vi "AH_ParseMSG.vi"(5 "InputMSG":string, 11 "error in (no error)":errorcluster) -> (2 "Cap Ind":string, 3 "Los Ind":string, 4 "Cap":dbl, 6 "Los":dbl, 8 "ExVolt":dbl, 10 "Error":i32, 15 "error out":errorcluster)   [LabVIEW 2021]
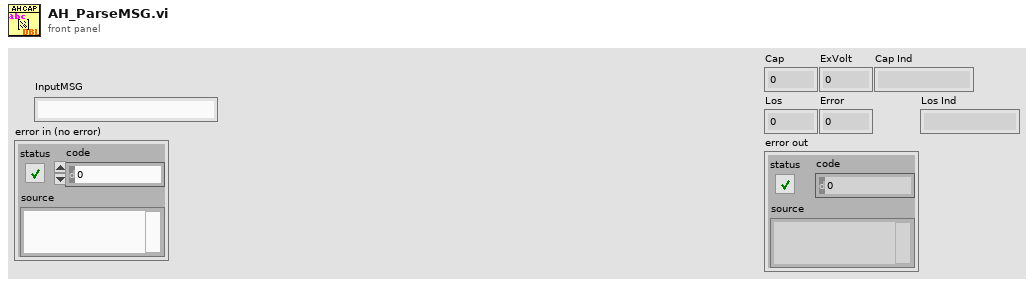
[diagram p1: front panel]
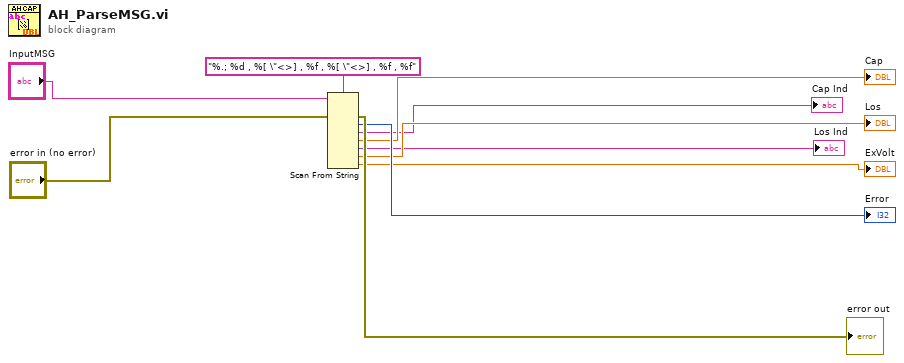
[diagram p0: block diagram]
diagram:
  n1 = Scan From String(format string="%.; %d , %[ \"<>] , %f , %[ \"<>] , %f , %f", input string="InputMSG", error in="error in (no error)") -> (error out=→"error out":errorcluster, output 1=→"Error":i32, output 2=→"Cap Ind":string, output 3=→"Cap":dbl, output 4=→"Los Ind":string, output 5=→"Los":dbl, output 6=→"ExVolt":dbl)  [unwired: 7 in, 2 out]
